vi "Parse Tags.vi"(8 "error in (no error)":errorcluster, 9 "[Tags]":string[](array[string]), 10 "[Control References]":refnum<vi>[](array[refnum]), 11 "Cluster of Controls":variant) -> (0 "error out":errorcluster, 1 "[Whole Tags]":string[](array[string]), 2 "[VData out]":variant[](array[variant]), 3 "[Parsed Tags]":T1[](array[typedef]))   [LabVIEW 2018]
doc: "Converts a variant cluster input and/or an array of references and/or an array of strings to an array of tag information as well as variant data.\nNote1: Empty variant data will be output for Array of Strings.\nNote2: The names/strings will be parsed for any text before the first space in order to find the tags\n\nIf an array of references is input, the VI uses these references to get tag names using the references controls' labels. \n\nIf a cluster of controls is input, each item in the cluster will be used for its label and value.\n\nIf just an array of strings is input, the string values will be used as tags and there will be void values output."
uses:
  Shared Controls/Parsed Tag Cluster.ctl
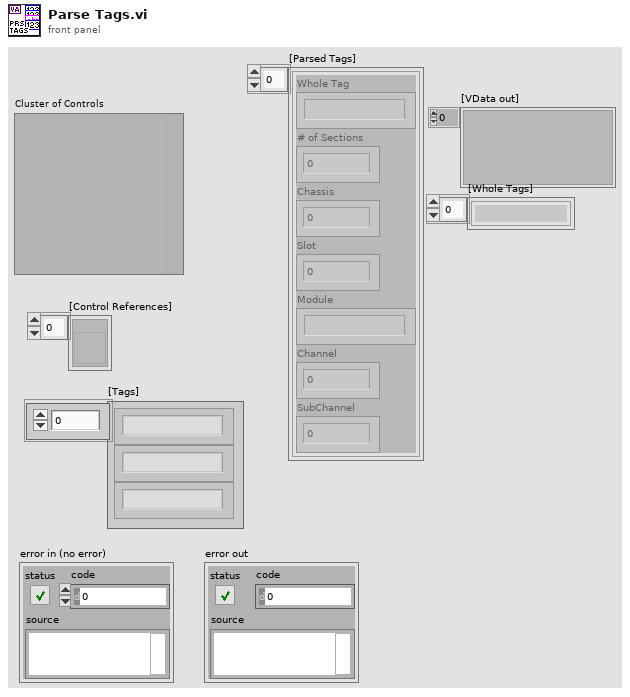
[diagram p1: front panel]
types:
  T1 = typedef "Parsed Tag Cluster.ctl" = cluster{"Whole Tag":string, "# of Sections":u8, "Chassis":u8, "Slot":u8, "Module":string, "Channel":u8, "SubChannel":u8}
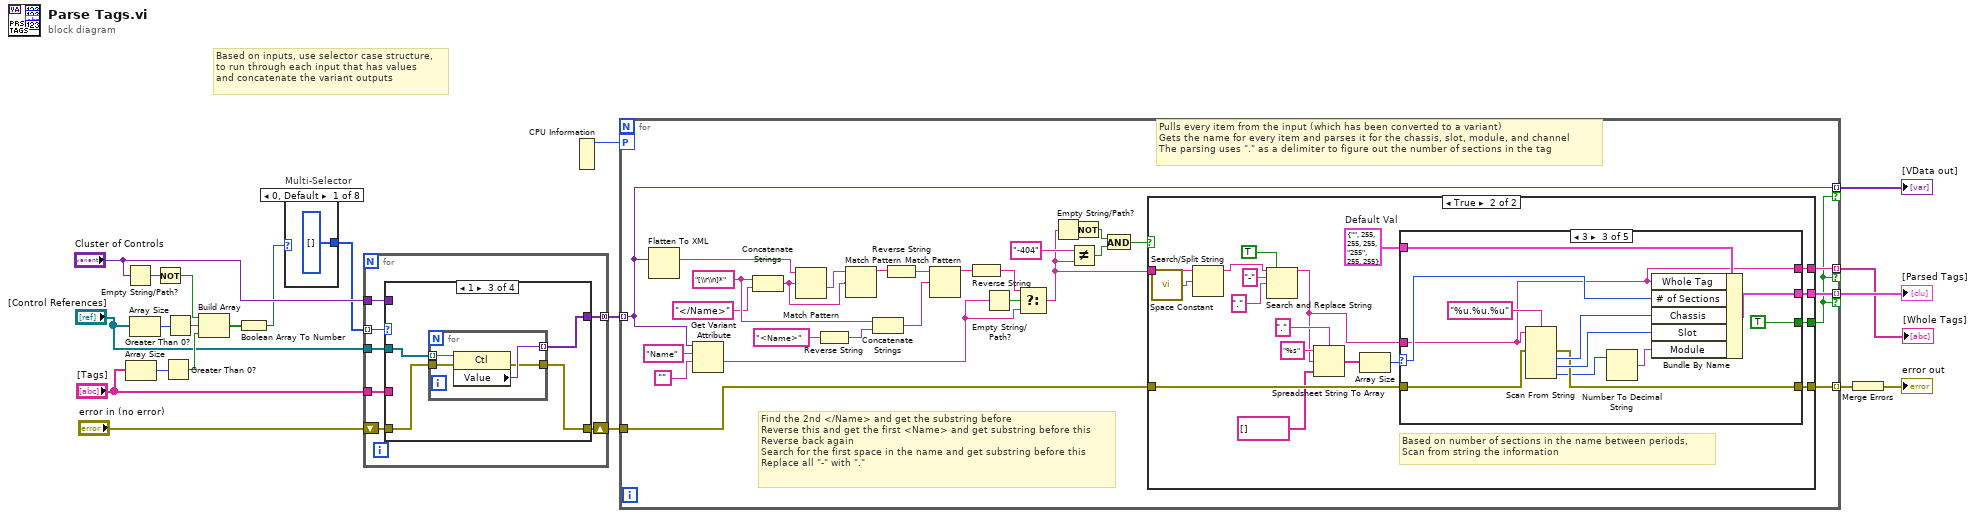
[diagram p0: block diagram]
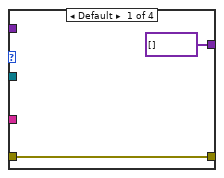
[diagram p2: hidden frame]
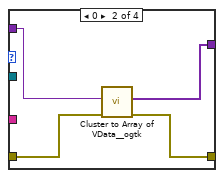
[diagram p3: hidden frame]
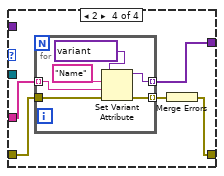
[diagram p4: hidden frame]
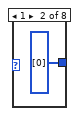
[diagram p5: hidden frame]
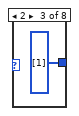
[diagram p6: hidden frame]
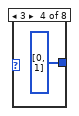
[diagram p7: hidden frame]
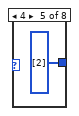
[diagram p8: hidden frame]
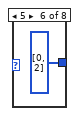
[diagram p9: hidden frame]
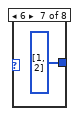
[diagram p10: hidden frame]
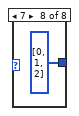
[diagram p11: hidden frame]
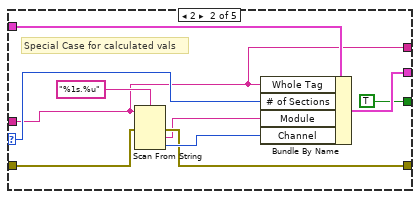
[diagram p14: hidden frame]
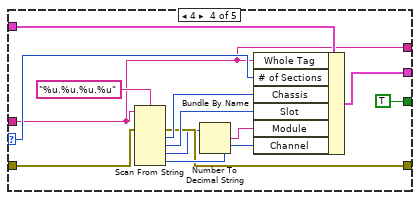
[diagram p15: hidden frame]
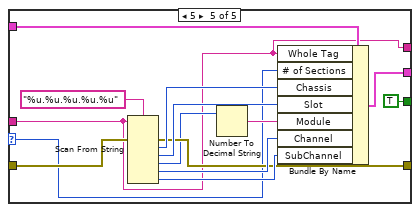
[diagram p16: hidden frame]
diagram:
  # "Based on inputs, use selector case structure,\nto run through each input that has values\nand concatenate the variant outputs"
  n1 = Empty String/Path?(string/path="Cluster of Controls") -> (empty?=w8:bool)
  n2 = Array Size(array="[Tags]") -> (size(s)=w14:i32)
  n3 = Array Size(array="[Control References]") -> (size(s)=w15:i32)
  n4 = Not(x=w8) -> (.not. x?=w7:bool)
  n5 = Greater Than 0?(x=w14) -> (x > 0?=w12:bool)
  n6 = Greater Than 0?(x=w15) -> (x > 0?=w13:bool)
  n7 = Build Array(w7, w13, w12) -> (w4:bool[])
  n8 = Boolean Array To Number(Boolean array=w4) -> (number=w6:u32)
  n9 = case "Multi-Selector" shown="0, Default" w6 {
    tunnel: [u32[] [] u32[] [0] u32[] [1] u32[] [0, 1] u32[] [2] u32[] [0, 2] u32[] [1, 2] u32[] [0, 1, 2]] -> w5
    frame 0, Default {
    }
    frame 1 {
    }
    frame 2 {
    }
    frame 3 {
    }
    frame 4 {
    }
    frame 5 {
    }
    frame 6 {
    }
    frame 7 {
    }
  }
  n10 = for {
    tunnel: [w36] -> w19 mode=concatenating
    tunnel: "[Control References]" -> [w33]
    tunnel: "[Tags]" -> [w32]
    tunnel: "Cluster of Controls" -> [w31]
    tunnel: w5 -> [w30] mode=indexing
    shift-right: [w34] -> w18
    shift-left: "error in (no error)" -> [w35]
    n11 = case shown="1" w30 {
      tunnel: [variant[] [] ("Array of VData") w42 w45 w55] -> w36
      tunnel: w35 -> [w37 w41 w44 w54]
      tunnel: [w37 w40 w43 w51] -> w34
      tunnel: w33 -> [_ _ w46 _]
      tunnel: w31 -> [_ w39 _ _]
      tunnel: w32 -> [_ _ _ w52]
      frame Default {
      }
      frame 0 {
        n12 = call <userlib>:"Cluster to Array of VData__ogtk.vi"("error in (no error)"=w41, "Cluster"=w39) -> ("error out"=w40:errorcluster, "Array of VData"=w42:variant[])  [unwired: 8 in]
      }
      frame 1 {
        n13 = for {
          tunnel: w46 -> [w50] mode=indexing
          tunnel: [w49] -> w45 mode=indexing
          tunnel: w44 -> [w48]
          tunnel: [w47] -> w43
          n14 = property class="Ctl"(reference=w50, error in=w48) -> (error out=w47:errorcluster, "Value"=w49:variant)  [unwired: 1 out]
        }
      }
      frame 2 {
        n15 = for {
          tunnel: [w58] -> w55 mode=indexing
          tunnel: w54 -> [w61]
          tunnel: [w60] -> w53 mode=indexing
          tunnel: w52 -> [w57] mode=indexing
          n16 = Set Variant Attribute(Variant=variant(string "TagOnly") ("variant"), name="Name", value=w57, error in=w61) -> (Variant out=w58:variant, error out=w60:errorcluster)  [unwired: 1 out]
        }
        n17 = Merge Errors(w53) -> (w51:errorcluster)
      }
    }
  }
  n18 = CPU Information() -> (4:w1:i32)  [unwired: 3 out]
  n19 = for {
    tunnel: [w87] -> w21 mode=indexing if=w68
    tunnel: w19 -> [w75] mode=indexing
    tunnel: w18 -> [w89]
    tunnel: [w88] -> w20 mode=indexing
    tunnel: [w75] -> w16 mode=indexing if=w68
    tunnel: [w69] -> w2 mode=indexing if=w68
    workers-P: w1 -> [_]
    w85 = "[\\r\\n]*"
    # "Find the 2nd </Name> and get the substring before\nReverse this and get the first <Name> and get substring before this\nReverse back again\nSearch for the first space in the name and get substring before this\nReplace all \"-\" with \".\""
    # "Pulls every item from the input (which has been converted to a variant)\nGets the name for every item and parses it for the chassis, slot, module, and channel\nThe parsing uses \".\" as a delimiter to figure out the number of sections in the tag"
    n20 = Flatten To XML(anything=w75) -> (xml string=w82:string)
    n21 = Get Variant Attribute(Variant=w75, name="Name", default value (empty Variant)="") -> (value=w70:string)  [unwired: 1 in, 3 out]
    n22 = Concatenate Strings(w85, "</Name>" ("Substring")) -> (w78:string)
    n23 = Match Pattern(string=w82, regular expression=w78) -> (after substring=w79:string)  [unwired: 1 in, 3 out]
    n24 = Reverse String(1:"<Name>") -> (0:w84:string)
    n25 = Match Pattern(string=w79, regular expression=w78) -> (before substring=w77:string)  [unwired: 1 in, 3 out]
    n26 = Concatenate Strings(w85, w84) -> (w86:string)
    n27 = Reverse String(1:w77) -> (0:w83:string)
    n28 = Match Pattern(string=w83, regular expression=w86) -> (before substring=w76:string)  [unwired: 1 in, 3 out]
    n29 = Reverse String(1:w76) -> (0:w71:string)
    n30 = Empty String/Path?(string/path=w70) -> (empty?=w72:bool)
    n31 = Select(t=w71, s=w72, f=w70) -> (s? t:f=w66:string)
    n32 = Empty String/Path?(string/path=w66) -> (empty?=w65:bool)
    n33 = Not Equal?(x="-404", y=w66) -> (x != y?=w64:bool)
    n34 = Not(x=w65) -> (.not. x?=w62:bool)
    n35 = And(x=w62, y=w64) -> (x .and. y?=w63:bool)
    n36 = case shown="True" w63 {
      tunnel: w89 -> [w90 w107]
      tunnel: [w90 w106] -> w88
      tunnel: [_ w105] -> w87
      tunnel: [_ w93] -> w69
      tunnel: [_ w92] -> w68
      tunnel: w66 -> [_ w91]
      frame False {
      }
      frame True {
        w108 = T1 {"Whole Tag"="", "# of Sections"=255, "Chassis"=255, "Slot"=255, "Module"="255", "Channel"=255, "SubChannel"=255}  # Default Val
        # "Based on number of sections in the name between periods,\nScan from string the information"
        n37 = call <vilib>:"Space Constant.vi"() -> ("String"=w94:string)
        n38 = Search/Split String(string=w91, search string/char (-)=w94) -> (substring before match=w95:string)  [unwired: 1 in, 2 out]
        n39 = Search and Replace String(replace all?=TRUE ("replace all? (F)"), input string=w95, search string="-", replace string="." ("replace string (\"\")")) -> (result string=w99:string)  [unwired: 4 in, 3 out]
        n40 = Spreadsheet String To Array(delimiter (Tab)=".", format string="%s", spreadsheet string=w99, array type (2D Dbl)=string[] []) -> (array=w103:string[])
        n41 = Array Size(array=w103) -> (size(s)=w102:i32)
        n42 = case shown="3" w102 {
          selector: w102 -> [_ w111 w121 w133 w146]
          tunnel: w108 -> [_ w117 w128 w140 w158]
          tunnel: w107 -> [w109 w115 w126 w138 w152]
          tunnel: [w109 w116 w127 w139 w151] -> w106
          tunnel: [_ w114 w123 w135 w147] -> w105
          tunnel: w99 -> [_ w110 w120 w132 w145]
          tunnel: [_ TRUE TRUE TRUE TRUE] -> w92
          tunnel: [_ w110 w120 w132 w145] -> w93
          frame Default {
          }
          frame 2 {
            # "Special Case for calculated vals"
            n43 = Scan From String(format string="%1s.%u" ("regular expression"), input string=w110, error in=w115) -> (error out=w116:errorcluster, output 1=w112:string, output 2=w118:u32)  [unwired: 3 in, 2 out]
            n44 = Bundle By Name(cluster=w117, "Whole Tag"=w110, "# of Sections"=w111, "Module"=w112, "Channel"=w118) -> (w114:T1)
          }
          frame 3 {
            n45 = Scan From String(format string="%u.%u.%u" ("regular expression"), input string=w120, error in=w126) -> (error out=w127:errorcluster, output 1=w130:u32, output 2=w129:u32, output 3=w125:u32)  [unwired: 4 in, 2 out]
            n46 = Number To Decimal String(number=w125) -> (decimal integer string=w124:string)  [unwired: 1 in]
            n47 = Bundle By Name(cluster=w128, "Whole Tag"=w120, "# of Sections"=w121, "Chassis"=w130, "Slot"=w129, "Module"=w124) -> (w123:T1)
          }
          frame 4 {
            n48 = Scan From String(format string="%u.%u.%u.%u" ("regular expression"), input string=w132, error in=w138) -> (error out=w139:errorcluster, output 1=w143:u32, output 2=w142:u32, output 3=w137:u32, output 4=w141:u32)  [unwired: 5 in, 2 out]
            n49 = Number To Decimal String(number=w137) -> (decimal integer string=w136:string)  [unwired: 1 in]
            n50 = Bundle By Name(cluster=w140, "Whole Tag"=w132, "# of Sections"=w133, "Chassis"=w143, "Slot"=w142, "Module"=w136, "Channel"=w141) -> (w135:T1)
          }
          frame 5 {
            n51 = Scan From String(format string="%u.%u.%u.%u.%u" ("regular expression"), input string=w145, error in=w152) -> (error out=w151:errorcluster, output 1=w156:u32, output 2=w155:u32, output 3=w150:u32, output 4=w154:u32, output 5=w153:u32)  [unwired: 6 in, 2 out]
            n52 = Number To Decimal String(number=w150) -> (decimal integer string=w149:string)  [unwired: 1 in]
            n53 = Bundle By Name(cluster=w158, "Whole Tag"=w145, "# of Sections"=w146, "Chassis"=w156, "Slot"=w155, "Module"=w149, "Channel"=w154, "SubChannel"=w153) -> (w147:T1)
          }
        }
      }
    }
  }
  "[Parsed Tags]" <- w21
  "[VData out]" <- w16
  "[Whole Tags]" <- w2
  n54 = Merge Errors(w20) -> (→"error out":errorcluster)
